vi "Robot Sound Player.vi"() -> ()   [LabVIEW 2015]
doc: "This VI illustrates how to play a sound file directly to the speakers. It uses Play Sound File.vi which opens a file and starts playing immediately and asynchronously (as opposed to the method shown in Sound File to Sound Output.vi example)."
panel:
  in  "Sound File Path":path=path "C:/Windows/Media/ringout.wav"
  in  "Stop":bool
  in  "Device ID":u32
  out "Sound Is Playing?":bool
  # "Overview: Demonstrates the use of the Sound Functions to play a sound file.\nInstructions:\n1. Specify the Device ID.\n2. Run the VI. It may take a several seconds to load the file and start playing the sound."
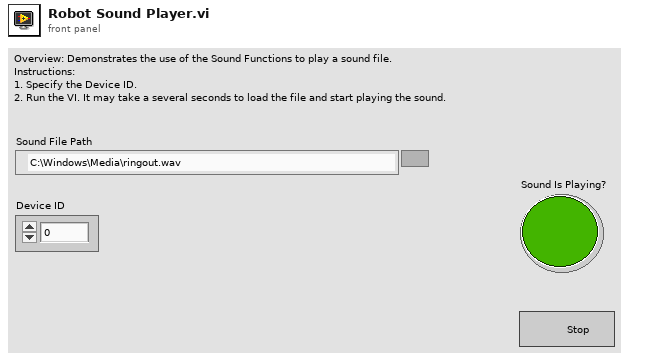
[diagram p1: front panel]
types:
  T1 = typedef "Sound Output Task ID.ctl" = u32
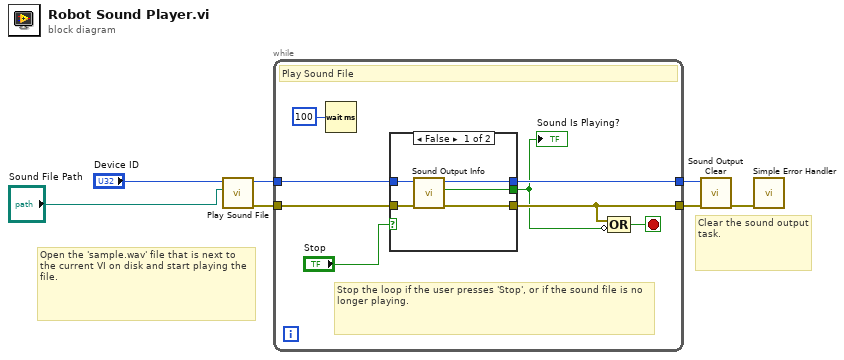
[diagram p0: block diagram]
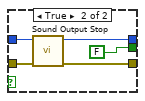
[diagram p2: hidden frame]
diagram:
  # "Clear the sound output task."
  # "Open the 'sample.wav' file that is next to the current VI on disk and start playing the file."
  n1 = call <vilib>:"Play Sound File.vi"("path"="Sound File Path", "device ID"="Device ID") -> ("error out"=w6:errorcluster, "task ID"=w7:T1)  [unwired: 8 in]
  n2 = while {
    tunnel: w7 -> [w9]
    tunnel: [w14] -> w4
    tunnel: w6 -> [w10]
    tunnel: [w13] -> w5
    stop <- w15 stop-if-true
    # "Stop the loop if the user presses 'Stop', or if the sound file is no longer playing."
    # "Play Sound File"
    n3 = Wait (ms)(milliseconds to wait=u32 100) -> ()  [unwired: 1 out]
    n4 = case shown="False" "Stop" {
      tunnel: w10 -> [w20 w24]
      tunnel: [w19 w22] -> w14
      tunnel: w9 -> [w18 w25]
      tunnel: [w17 w23] -> w13
      tunnel: [w16 FALSE] -> w12
      frame False {
        n5 = call <vilib>:"Sound Output Info.vi"("error in (no error)"=w20, "task ID"=w18) -> ("error out"=w17:errorcluster, "is playing?"=w16:bool, "task ID out"=w19:T1)  [unwired: 6 in, 1 out]
      }
      frame True {
        n6 = call <vilib>:"Sound Output Stop.vi"("error in (no error)"=w24, "task ID"=w25) -> ("error out"=w23:errorcluster, "task ID out"=w22:T1)  [unwired: 8 in]
      }
    }
    "Sound Is Playing?" <- w12
    n7 = Compound Arithmetic op=OR(w13, invert w12) -> (w15:bool)
  }
  n8 = call <vilib>:"Sound Output Clear.vi"("error in (no error)"=w5, "task ID"=w4) -> ("error out"=w2:errorcluster)  [unwired: 9 in]
  n9 = call <vilib>:"Simple Error Handler.vi"("error in (no error)"=w2) -> ()  [unwired: 4 in, 5 out]
